vi "SaveLoadMotorConfig.vi"(10 "Save? (F)":bool, 11 "MotorConfig(in)":T1={"Offset"={"Magnet Z"=10.0, "Magnet rotation"=0.0, "Camera"={"X"=0.0, "Y"=0.0}, "Piezo XY"={"X"=0.0, "Y"=0.0}, "Piezo Z"=0.0, "Coil XY"={"X"=0.0, "Y"=0.0}}, "Maximum pos"={"Magnet Z"=0.0, "Magnet rotation"=0.0, "Camera"={"X"=0.0, "Y"=0.0}, "Piezo XY"={"X"=0.0, "Y"=0.0}, "Piezo Z"=0.0, "Coil XY"={"X"=0.0, "Y"=0.0}}, "Min limited?"={"Magnet Z"=FALSE, "Magnet rotation"=FALSE, "Camera"={"X"=FALSE, "Y"=FALSE}, "Piezo XY"={"X"=FALSE, "Y"=FALSE}, "Piezo Z"=FALSE, "Coil XY"={"X"=FALSE, "Y"=FALSE}}, "Max limited?"={"Magnet Z"=FALSE, "Magnet rotation"=FALSE, "Camera"={"X"=FALSE, "Y"=FALSE}, "Piezo XY"={"X"=FALSE, "Y"=FALSE}, "Piezo Z"=FALSE, "Coil XY"={"X"=FALSE, "Y"=FALSE}}, "Has velocity support"={"Magnet Z"=FALSE, "Magnet rotation"=FALSE, "Camera"={"X"=FALSE, "Y"=FALSE}, "Piezo XY"={"X"=FALSE, "Y"=FALSE}, "Piezo Z"=FALSE, "Coil XY"={"X"=FALSE, "Y"=FALSE}}, "Default velocity"={"Magnet Z"=0.0, "Magnet rotation"=0.0, "Camera"={"X"=0.0, "Y"=0.0}, "Piezo XY"={"X"=0.0, "Y"=0.0}, "Piezo Z"=0.0, "Coil XY"={"X"=0.0, "Y"=0.0}}}) -> (1 "No error?":bool, 2 "motor config file":path, 3 "MotorConfig":T1)   [LabVIEW 2011]
uses:
  MotorConfigType.ctl
  MotorPosType.ctl
  Typedefs/XYf.ctl
  MotorPosFlagsType.ctl
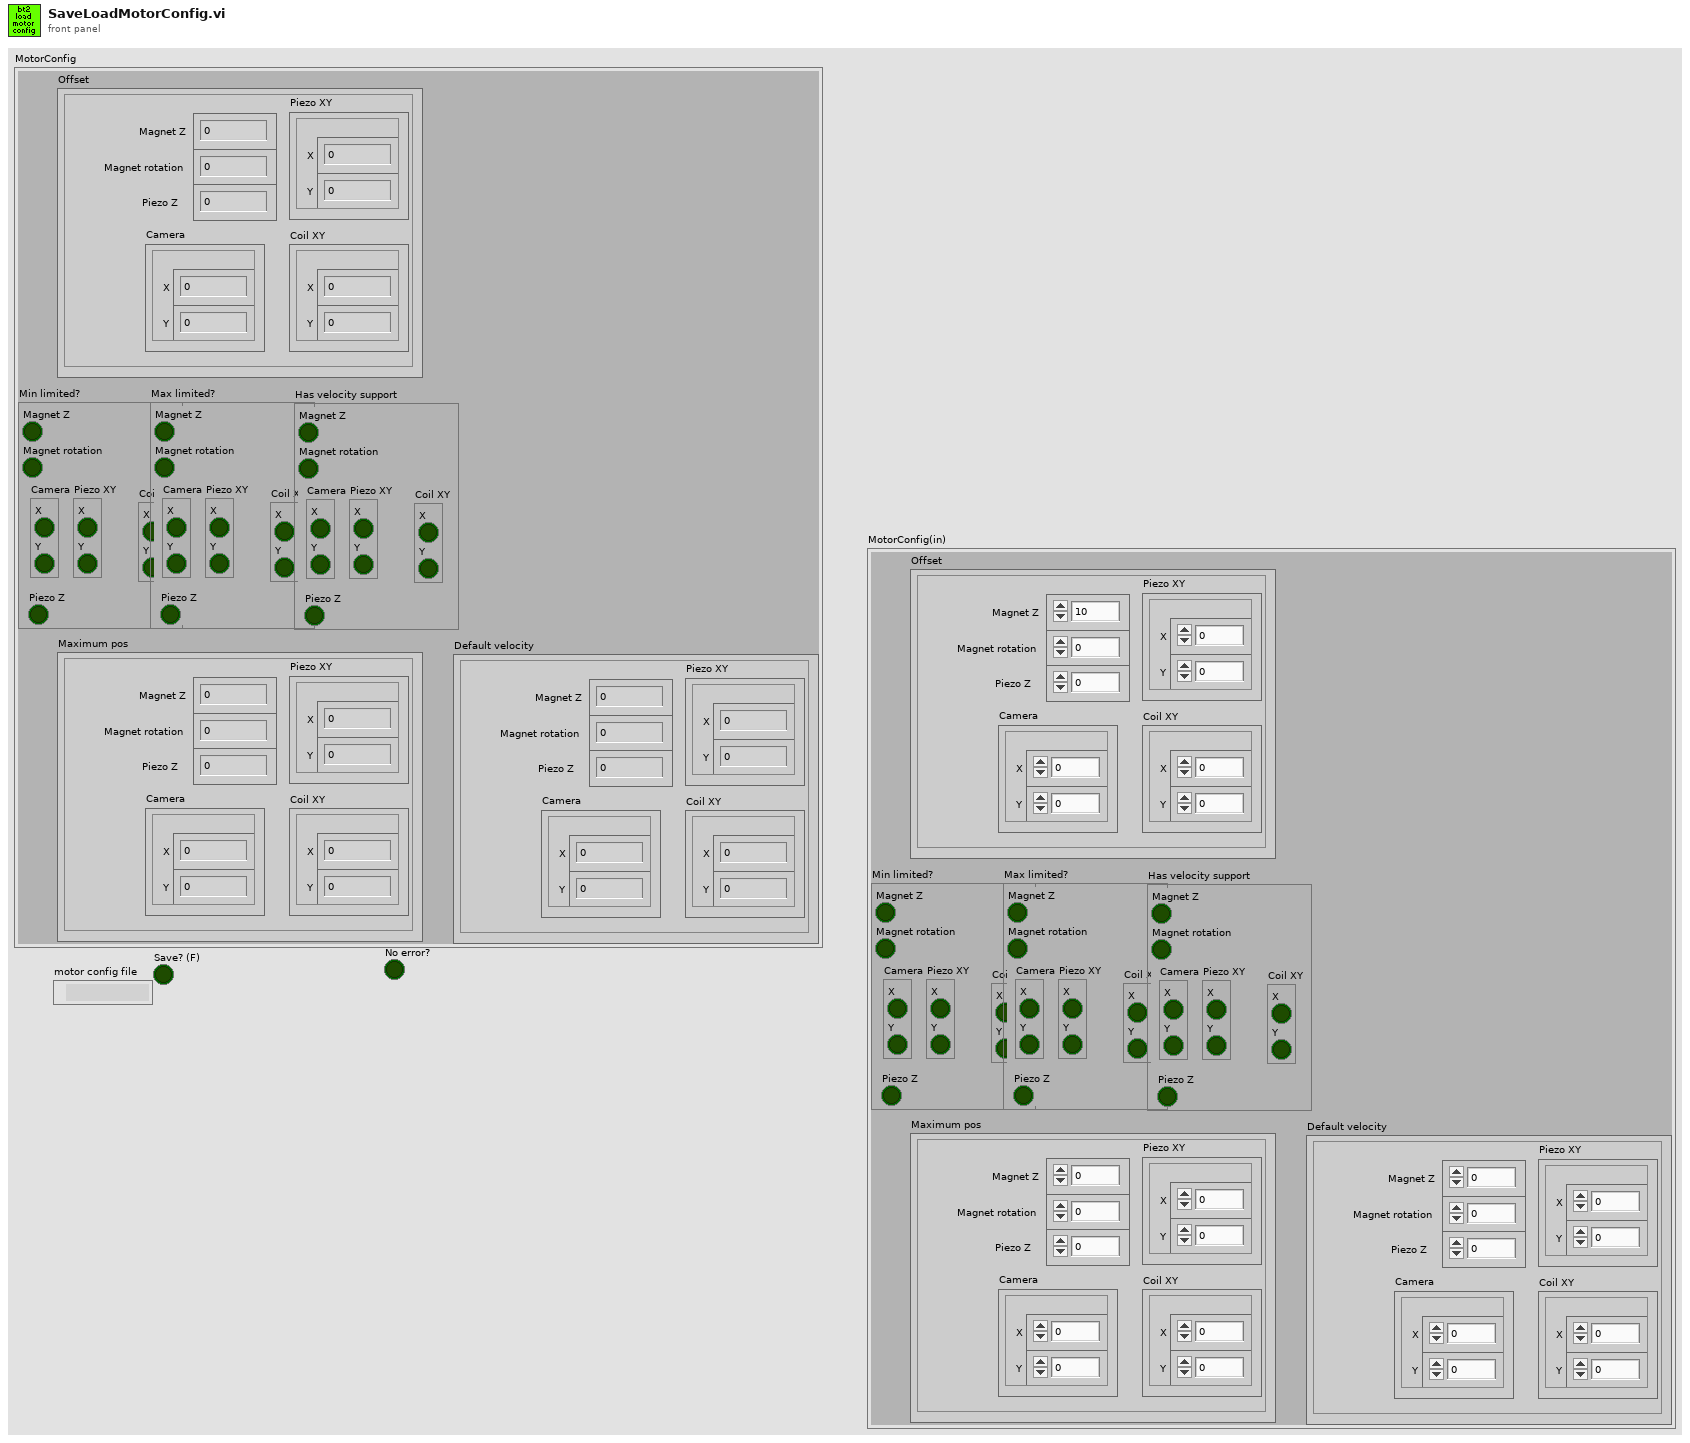
[diagram p1: front panel]
types:
  T1 = typedef "MotorConfigType.ctl" = cluster{"Offset":T2, "Maximum pos":T2, "Min limited?":T4, "Max limited?":T4, "Has velocity support":T4, "Default velocity":T2}
  T2 = typedef "MotorPosType.ctl" = cluster{"Magnet Z":dbl, "Magnet rotation":dbl, "Camera":T3, "Piezo XY":T3, "Piezo Z":dbl, "Coil XY":T3}
  T3 = typedef "XYf.ctl" = cluster{"X":sgl, "Y":sgl}
  T4 = typedef "MotorPosFlagsType.ctl" = cluster{"Magnet Z":bool, "Magnet rotation":bool, "Camera":cluster{"X":bool, "Y":bool}, "Piezo XY":cluster{"X":bool, "Y":bool}, "Piezo Z":bool, "Coil XY":cluster{"X":bool, "Y":bool}}
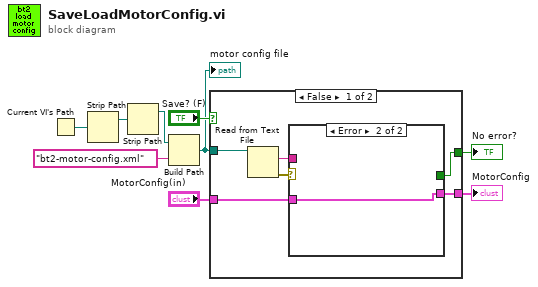
[diagram p0: block diagram]
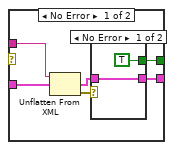
[diagram p2: hidden frame]
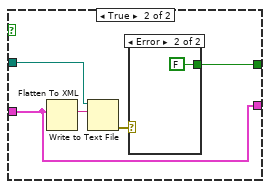
[diagram p4: hidden frame]
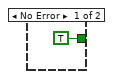
[diagram p5: hidden frame]
diagram:
  n1 = Current VI's Path() -> (path=w6:path)
  n2 = Strip Path(path=w6) -> (stripped path=w7:path)  [unwired: 1 out]
  n3 = Strip Path(path=w7) -> (stripped path=w8:path)  [unwired: 1 out]
  n4 = Build Path(base path=w8, name or relative path="bt2-motor-config.xml") -> (appended path=w2:path)
  "motor config file" <- w2
  n5 = case shown="False" "Save? (F)" {
    tunnel: [w15 w26] -> w9
    tunnel: w2 -> [w11 w29]
    tunnel: [w12 w27] -> w4
    tunnel: "MotorConfig(in)" -> [w10 w26]
    frame False {
      n6 = Read from Text File(file (use dialog)=w11) -> (text=w14:string, error out=w13:errorcluster)  [unwired: 3 in, 2 out]
      n7 = case shown="Error" w13 {
        tunnel: w10 -> [w21 w25]
        tunnel: w14 -> [w20 _]
        tunnel: [w17 w25] -> w15
        tunnel: [w16 _] -> w12
        frame No Error {
          n8 = Unflatten From XML(xml string=w20, type=w21) -> (value=w19:T1, error out=w18:errorcluster)  [unwired: 1 in]
          n9 = case shown="No Error" w18 {
            tunnel: w19 -> [w23 w24]
            tunnel: [w23 w24] -> w17
            tunnel: [TRUE _] -> w16
            frame No Error {
            }
            frame Error {
            }
          }
        }
        frame Error {
        }
      }
    }
    frame True {
      n10 = Flatten To XML(anything=w26) -> (xml string=w30:string)
      n11 = Write to Text File(file (use dialog)=w29, text=w30) -> (error out=w28:errorcluster)  [unwired: 2 in, 2 out]
      n12 = case shown="Error" w28 {
        tunnel: [TRUE FALSE] -> w27
        frame No Error {
        }
        frame Error {
        }
      }
    }
  }
  "MotorConfig" <- w9
  "No error?" <- w4
